vi "Query 2614 output state.vi"(0 "VISA resource name":refnum<visa-resource-name>, 5 "Source Measure Unit Channel (0: Channel A)":i32(ring) items=["Channel A", "Channel B"], 11 "error in (no error)":errorcluster) -> (4 "VISA resource name out":refnum<visa-resource-name>, 6 "levelv":dbl, 15 "error out":errorcluster)   [LabVIEW 2019, in "User lib.lvlib"]
doc: "Configures the source level."
uses:
  User lib.lvlib
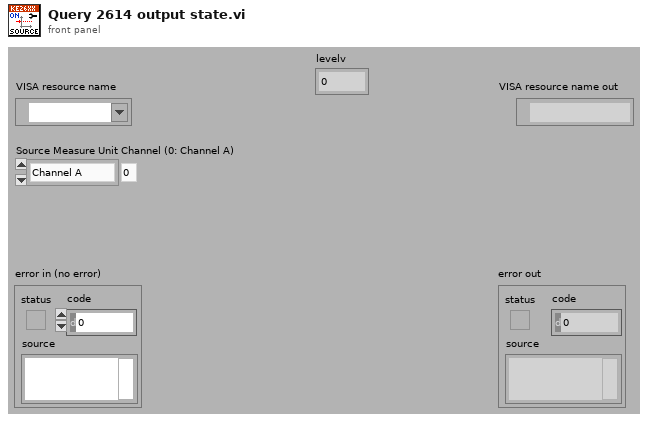
[diagram p1: front panel]
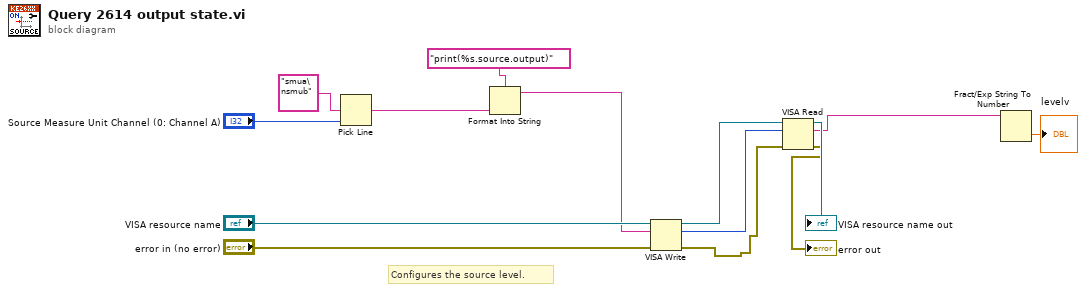
[diagram p0: block diagram]
diagram:
  # "Configures the source level."
  n1 = Pick Line(multi-line string="smua\nsmub", line index="Source Measure Unit Channel (0: Channel A)") -> (output string=w10:string)  [unwired: 1 in]
  n2 = Format Into String(format string="print(%s.source.output)", w10) -> (resulting string=w9:string)  [unwired: 2 in, 1 out]
  n3 = VISA Write(VISA resource name="VISA resource name", write buffer=w9, error in (no error)="error in (no error)") -> (VISA resource name out=w7:refnum<visa-resource-name>, return count=w5:u32, error out=w6:errorcluster)
  n4 = VISA Read(VISA resource name=w7, byte count=w5, error in (no error)=w6) -> (VISA resource name out=→"VISA resource name out":refnum<visa-resource-name>, read buffer=w2:string, error out=→"error out":errorcluster)  [unwired: 1 out]
  n5 = Fract/Exp String To Number(string=w2) -> (number=→"levelv":dbl)  [unwired: 3 in, 1 out]
